vi "Curtin1_DAQ.vi"(8 "error in (no error)":errorcluster) -> (1 "Buffer":T3, 3 "Tap":T2)   [LabVIEW 2022 SP3]
uses:
  <extravilib>/ChannelInstances/Tag-a[.](wfm(dbl)).lvlib
  Mic_Global.vi
  <extravilib>/ChannelInstances/Tag-a[.](wfm(dbl))/))Channel.ctl
  <extravilib>/ChannelInstances/Lossy Stream-a[.](wfm(dbl))/)Channel.ctl
  <extravilib>/ChannelInstances/Lossy Stream-a[.](wfm(dbl)).lvlib
  PreferencesControl.ctl
panel:
  out "Settings":T1={"Name of test"="", "Date"=timestamp(0 s since 1904-01-01), "Location"="", "Template"="", "Soundcard"="", "resolution"=32, "Sampling rate"=48000, "Ch1 Gain "=25.0, "Ch2 Gain"=10.0, "Sample time (s)"=0.3, "Pre-trigger (s)"=0.01, "Hammer Threshold"=10.0, "Positions"=12, "Taps/Position"=5, "Set Names"="", "Freq resolution"=10.0, "Hammer cutoff"=0.0, "Mic cutoff"=0.0, "Double bounce "=0.0, "Hammer Cal"=10.0, "dB Offset"=0.0, "Accel Cal"=10.0, "Vibrometer Cal"=0.0, "Mic Cal"=1.0, "Output"=2, "Voltage Cal"=1.0, "Vibrometer Port"="ASRL27::INSTR", "Range"=4, "High Pass"=2, "Bandwidth"=4, "X Range"=[], "Y Range"=[], "dB Spread"=0.0, "Trigger"=0, "Ch_1"=25, "Ch_2"=25, "flip?"=FALSE, "60Hz"=FALSE, "Time offset"=0.0, "Piezo Cal"=1.0, "Default Notes"=""} {"Ch_2" min=1 step=1; "Ch_1" min=1 max=100 step=1; "Trigger" items=["Hammer (force)", "Self-tap", "Spacebar"]; "Bandwidth" items=["1 kHz"=1, "5 kHz"=5, "10 kHz"=10, "25 kHz"=25, "50 kHz"=50, "100 kHz"=100]; "High Pass" items=["Off", "13 Hz", "104 Hz"]; "Range" items=["10 mm/s"=1, "20 mm/s"=2, "50 mm/s"=5, "100 mm/s"=10, "200 mm/s"=20, "500 mm/s"=50, "1 m/s"=100, "2 m/s"=200]; "Output" items=["Accelerometer", "Speed (from acceleration)", "Microphone", "Vibrometer", "Piezo"]; "Voltage Cal" format="%#_13g"; "Ch2 Gain" format="%#_13g"; "Ch1 Gain" format="%#_13g"; "Double bounce" min=0.0; "Mic cutoff" min=0.0 format="%#_4g"; "Hammer cutoff" min=0.0 format="%#_4g"; "Freq resolution" min=0.0; "Pre-trigger (s)" format="%#_13g"; "Date" format="%<%H:%M\n%d/%m/%y>T"; "resolution" items=["16 bit"=16, "24 bit"=24, "32 bit"=32]; "Sampling rate" items=["22050 samp/s"=22050, "44100 samp/s"=44100, "48000 samp/s"=48000]}
  out "Microphone":waveform(dbl)(graph)
  out "Hammer":waveform(dbl)(graph)
  out "Task":T4(ring)=enum."Free run"
  in  "stop":bool
  # "Hz"
  # "dB"
  # "dB"
  # "sec"
  # "sec"
  # "mV/Pa"
  # "mV/m/s2"
  # "mV/mm/s"
  # "V/N"
  # "sec"
  # "sec"
  # "mV/N"
  # "a.u."
  # "a.u."
  # "sec"
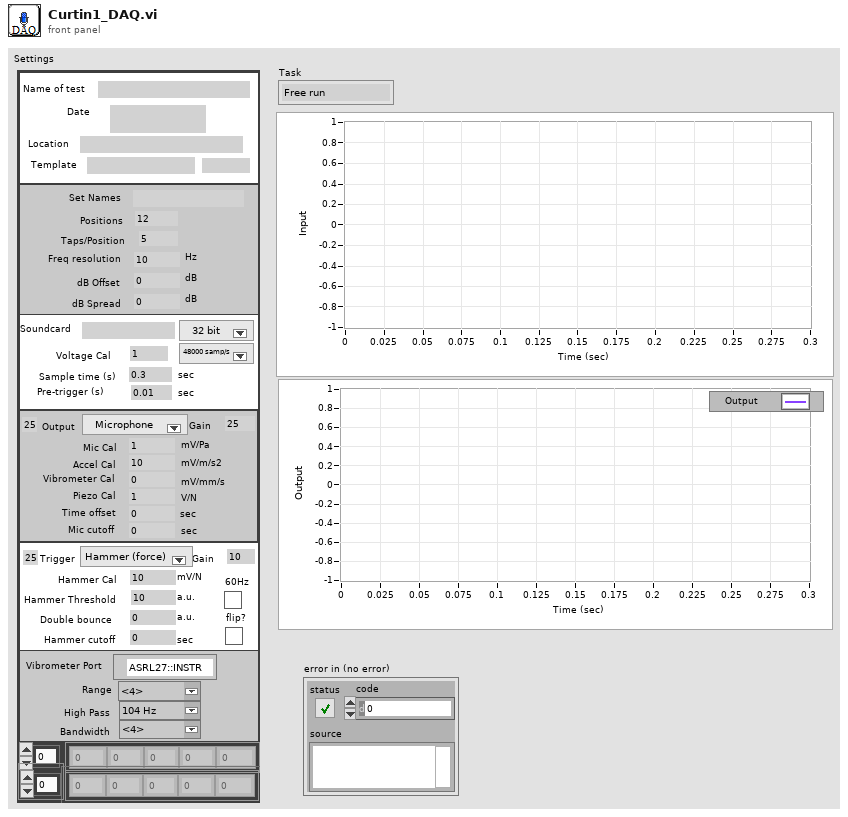
[diagram p1: front panel]
types:
  T1 = typedef "PreferencesControl.ctl" = cluster{"Name of test":string, "Date":timestamp, "Location":string, "Template":string, "Soundcard":string, "resolution":u16, "Sampling rate":u16, "Ch1 Gain ":dbl, "Ch2 Gain":dbl, "Sample time (s)":dbl, "Pre-trigger (s)":dbl, "Hammer Threshold":dbl, "Positions":i16, "Taps/Position":i16, "Set Names":string, "Freq resolution":dbl, "Hammer cutoff":dbl, "Mic cutoff":dbl, "Double bounce ":dbl, "Hammer Cal":dbl, "dB Offset":dbl, "Accel Cal":dbl, "Vibrometer Cal":dbl, "Mic Cal":dbl, "Output":u16, "Voltage Cal":dbl, "Vibrometer Port":refnum<visa-resource-name>, "Range":u16, "High Pass":u16, "Bandwidth":u16, "X Range":cluster{"Minimum":dbl, "Maximum":dbl, "Increment":dbl, "Minor Increment":dbl, "Start":dbl}[], "Y Range":cluster{"Minimum":dbl, "Maximum":dbl, "Increment":dbl, "Minor Increment":dbl, "Start":dbl}[], "dB Spread":dbl, "Trigger":u16, "Ch_1":u8, "Ch_2":u8, "flip?":bool, "60Hz":bool, "Time offset":dbl, "Piezo Cal":dbl, "Default Notes":string}
  T2 = typedef "Lossy Stream-a[.](wfm(dbl)).lvlib/)Channel.ctl" = refnum<queue>
  T3 = typedef "Tag-a[.](wfm(dbl)).lvlib/))Channel.ctl" = refnum<queue>
  T4 = enum16{"Initialize", "Free run", "One Shot - waiting", "One Shot - triggered", "Wait", "Close"}
  T5 = cluster{"task in":refnum<k21>, "Num Pts":i32, "timeout":dbl, "FIFO":i32, "Double Bounce":dbl, "Sensitivity (V/X)":dbl[]}
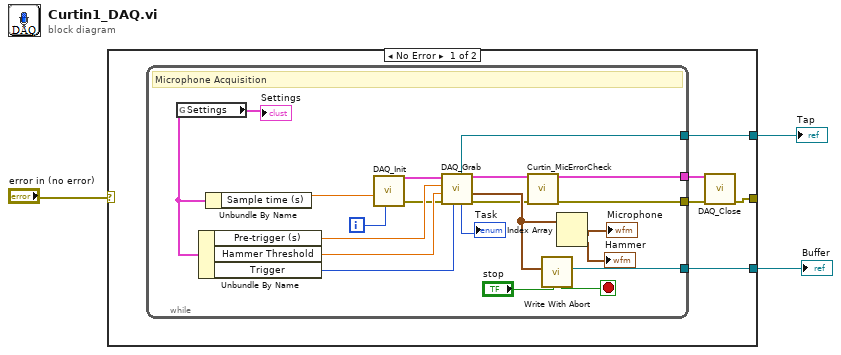
[diagram p0: block diagram]
diagram:
  n1 = case shown="No Error" "error in (no error)" {
    tunnel: [w7 _] -> w3
    tunnel: [w6 _] -> w1
    tunnel: [w4 _] -> _
    frame No Error {
      n2 = while {
        tunnel: [w26] -> w7
        tunnel: [w25] -> w8
        tunnel: [w19] -> w6
        tunnel: [w9] -> w5
        i -> [w14]
        stop <- w22 stop-if-true
        # "Microphone Acquisition"
        n3 = global read "Mic_Global.vi" "Settings"() -> (w15:T1)
        "Settings" <- w15
        n4 = Unbundle By Name(w15) -> ("Pre-trigger (s)"=w21:dbl, "Hammer Threshold"=w20:dbl, "Trigger"=w10:u16)
        n5 = Unbundle By Name(w15) -> ("Sample time (s)"=w16:dbl)
        n6 = call "DAQ_Init.vi"("itteration"=w14, "Sample time"=w16) -> ("error out"=w18:errorcluster, "DAQ Prams"=w17:T5)  [unwired: 8 in]
        n7 = call "DAQ_Grab.vi"("Input"=w10, "error In"=w18, "Threshold"=w20, "Pre-trigger (s)"=w21, "DAQ Prams"=w17) -> ("error out"=w9:errorcluster, "Buffer"=w24:waveform(dbl)[], "DAQ Prams"=w25:T5, "Start Task"=→"Task":T4, "Tap"=w19:T2)  [unwired: 1 in, 1 out]
        n8 = call "Curtin_MicErrorCheck.vi"("error in (no error)"=w9) -> ()  [unwired: 11 in]
        n9 = call <extravilib>:"Write With Abort.vi"("abort"="stop", "element"=w24) -> ("channel"=w26:T3, "aborted?"=w22:bool)  [unwired: 7 in, 1 out]
        n10 = Index Array(array=w24) -> (element #1=→"Microphone":waveform(dbl), element #2=→"Hammer":waveform(dbl))  [unwired: 2 in]
      }
      n11 = call "DAQ_Close.vi"("error in (no error)"=w5, "DAQ Prams"=w8) -> ("error out"=w4:errorcluster)  [unwired: 9 in]
    }
    frame Error {
    }
  }
  "Buffer" <- w3
  "Tap" <- w1
